vi "Set File IO Loop References.vi"(7 "File Loop Data in":T1, 8 "error in":errorcluster, 11 "call chain":string[](array[string])) -> (0 "error out":errorcluster, 2 "File Loop Data out":T1)   [LabVIEW 2018]
uses:
  Type Defs/File IO Loop Data.ctl
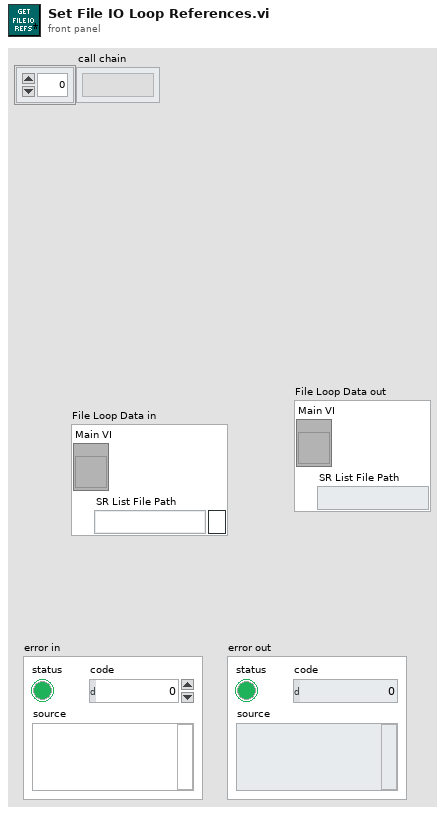
[diagram p1: front panel]
types:
  T1 = typedef "File IO Loop Data.ctl" = cluster{"Main VI":refnum<vi>, "SR List File Path":path}
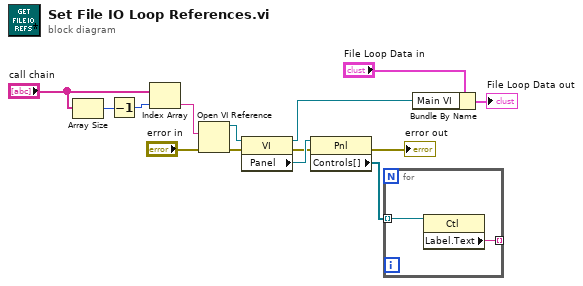
[diagram p0: block diagram]
diagram:
  n1 = Array Size(array="call chain") -> (size(s)=w6:i32)
  n2 = Decrement(x=w6) -> (x-1=w7:i32)
  n3 = Index Array(array="call chain", index=w7) -> (element=w8:string)
  n4 = Open VI Reference(vi path=w8, error in (no error)="error in") -> (vi reference=w13:refnum<vi>, error out=w10:errorcluster)  [unwired: 4 in]
  n5 = property class="VI"(reference=w13, error in=w10) -> (reference out=w4:refnum<vi>, error out=w11:errorcluster, "Panel"=w12:refnum<vi>)
  n6 = property class="Pnl"(reference=w12, error in=w11) -> (error out=→"error out":errorcluster, "Controls[]"=w9:refnum<vi>[])  [unwired: 1 out]
  n7 = for {
    tunnel: w9 -> [w16] mode=indexing
    tunnel: [w15] -> _ mode=indexing
    n8 = property class="Ctl"(reference=w16) -> ("Label.Text"=w15:string)  [unwired: 1 in, 2 out]
  }
  n9 = Bundle By Name(cluster="File Loop Data in", "Main VI"=w4) -> (→"File Loop Data out":T1)
